vi "Add User Friendly Error Text.vi"(7 "Force User Error":bool, 8 "error in (no error)":errorcluster, 10 "user error code":i32, 11 "User Error Message":string) -> (0 "error out":errorcluster, 3 "Error Text":string)   [LabVIEW 2018]
doc: "If error in contains an error, this vi modifies the error according to whether it is running in the development environment or as an executable. \n\nFor development environment: passes the error code through and appends the user message and user code as text in the source portion of the error cluster. \n\nFor an executable: the user code is used and the error in text is appended to the user message text for the source part of the error cluster.\n\nBy Mink Hollow Systems\nhttp://www.minkhollowsystems.com"
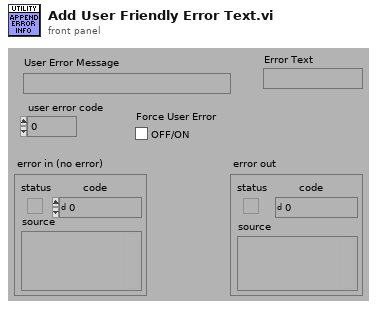
[diagram p1: front panel]
types:
  T1 = enum32{"invalid app kind", "Development System", "Run Time System", "Student Edition", "Embedded LabVIEW", "Evaluation", "Custom"}
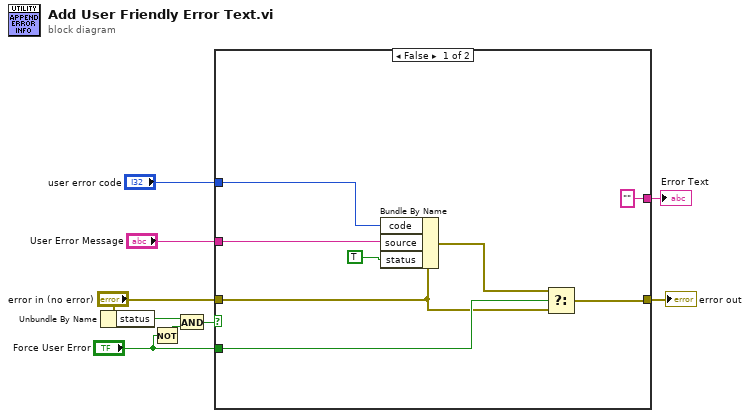
[diagram p0: block diagram]
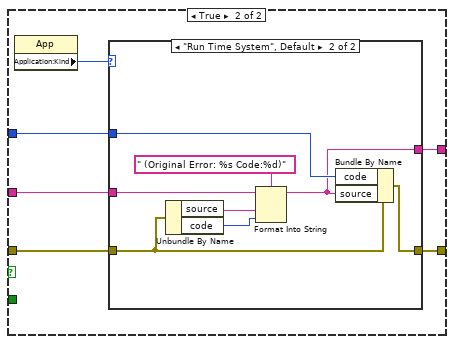
[diagram p2: hidden frame]
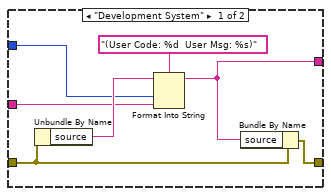
[diagram p3: hidden frame]
diagram:
  n1 = Unbundle By Name("error in (no error)") -> ("status"=w5:bool)
  n2 = Not(x="Force User Error") -> (.not. x?=w1:bool)
  n3 = And(x=w5, y=w1) -> (x .and. y?=w4:bool)
  n4 = case shown="False" w4 {
    tunnel: [w13 w22] -> w9
    tunnel: "User Error Message" -> [w11 w21]
    tunnel: "user error code" -> [w12 w20]
    tunnel: ["" w19] -> w6
    tunnel: "error in (no error)" -> [w14 w18]
    tunnel: "Force User Error" -> [w16 _]
    frame False {
      n5 = Bundle By Name(cluster=w14, "code"=w12, "source"=w11, "status"=TRUE) -> (w15:errorcluster)
      n6 = Select(t=w15, s=w16, f=w14) -> (s? t:f=w13:errorcluster)
    }
    frame True {
      n7 = property class="App"() -> ("Application:Kind"=w23:T1)  [unwired: 2 in, 2 out]
      n8 = case shown="\"Run Time System\", Default" w23 {
        tunnel: w18 -> [w28 w38]
        tunnel: [w27 w33] -> w22
        tunnel: w21 -> [w25 w37]
        tunnel: w20 -> [w26 w32]
        tunnel: [w24 w31] -> w19
        frame "Development System" {
          n9 = Unbundle By Name(w28) -> ("source"=w29:string)
          n10 = Format Into String(format string="(User Code: %d  User Msg: %s)", initial string=w29, w26, w25) -> (resulting string=w24:string)  [unwired: 1 in, 1 out]
          n11 = Bundle By Name(cluster=w28, "source"=w24) -> (w27:errorcluster)
        }
        frame "Run Time System", Default {
          n12 = Unbundle By Name(w38) -> ("source"=w35:string, "code"=w34:i32)
          n13 = Format Into String(format string=" (Original Error: %s Code:%d)", initial string=w37, w35, w34) -> (resulting string=w31:string)  [unwired: 1 in, 1 out]
          n14 = Bundle By Name(cluster=w38, "code"=w32, "source"=w31) -> (w33:errorcluster)
        }
      }
    }
  }
  "error out" <- w9
  "Error Text" <- w6
